vi "EpromCheckSameValue.vi"() -> ()   [LabVIEW 2016]
uses:
  <userlib>/ICNC/ICNC2.lvlib
panel:
  in  "Numeric 2":i32=1
  out "Numeric":i32
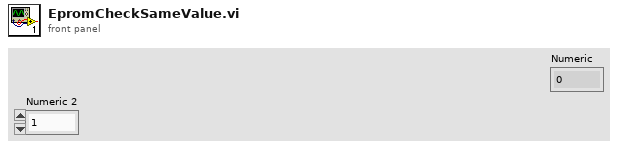
[diagram p1: front panel]
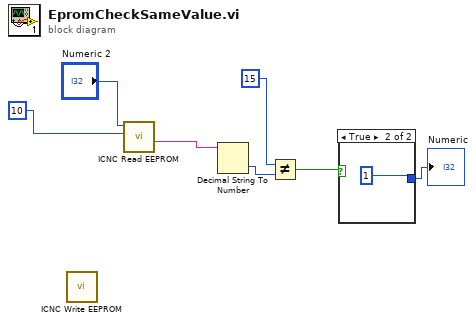
[diagram p0: block diagram]
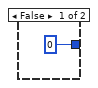
[diagram p2: hidden frame]
diagram:
  n1 = call <menus>:"ICNC Write EEPROM.vi"() -> ()  [unwired: 9 in, 3 out]
  n2 = call <menus>:"ICNC Read EEPROM.vi"("Length"=10, "StartAdress"="Numeric 2") -> ("Value out"=w4:string)  [unwired: 7 in, 2 out]
  n3 = Decimal String To Number(string=w4) -> (number=w3:i32)  [unwired: 2 in, 1 out]
  n4 = Not Equal?(x=15, y=w3) -> (x != y?=w2:bool)
  n5 = case shown="True" w2 {
    tunnel: [0 1] -> w1
    frame False {
    }
    frame True {
    }
  }
  "Numeric" <- w1
